vi "EditOptions.vi"(8 "error in":errorcluster, 11 "node in":refnum<class "CustomDevice.lvclass">) -> (0 "error out":errorcluster, 1 "edit options":T1, 2 "subnodes class":T2, 3 "node out":refnum<class "CustomDevice.lvclass">)   [LabVIEW 2019, in "CustomDevice.lvclass"]
doc: "Contains the options for the Menu that will be displayed when doing right click on an item.\nThe sub nodes class configures which nodes can be added to this nodes\nAnd the edit options determine which options are available for the node.\nThis configuration is stored in this VI in case some dynamic configuration is required for the menu options or sub nodes."
uses:
  CustomDevice.lvclass
  C:/Program Files (x86)/National Instruments/LabVIEW 2019/vi.lib/NI/Configuration Framework/Node/NISE_CEF_Node.lvclass
  <vilib>/NI/Configuration Framework/Node/SubNodeCluster.ctl
  <vilib>/NI/Configuration Framework/Node/NodeMenuOptions.ctl
  <vilib>/NI/Configuration Framework/Node/NISE_CEF_Node.lvclass/NISE_CEF_Node.ctl
  <vilib>/NI/Configuration Framework/Node/ReadChildren.vi
  <vilib>/NI/Configuration Framework/Node/ReadNodeClass.vi
  <vilib>/NI/Configuration Framework/Node/NISE_CEF_Node.lvclass
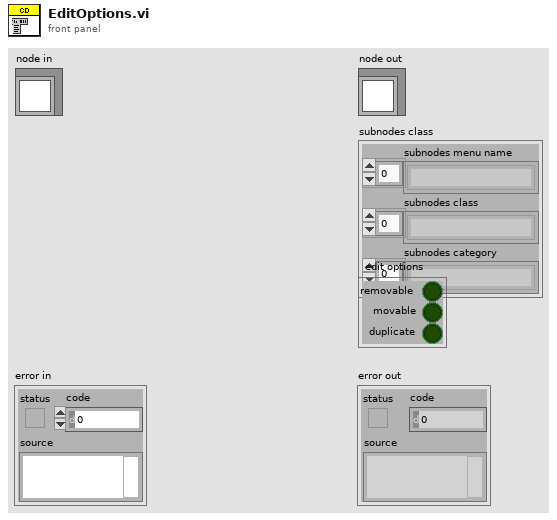
[diagram p1: front panel]
types:
  T1 = typedef "NISE_CEF_Node.lvclass/NodeMenuOptions.ctl" = cluster{"removable":bool, "movable":bool, "duplicate":bool}
  T2 = typedef "NISE_CEF_Node.lvclass/SubNodeCluster.ctl" = cluster{"subnodes menu name":string[], "subnodes class":string[], "subnodes category":string[]}
  T3 = typedef "NISE_CEF_Node.lvclass/NodeRef.ctl" = refnum<data-value>
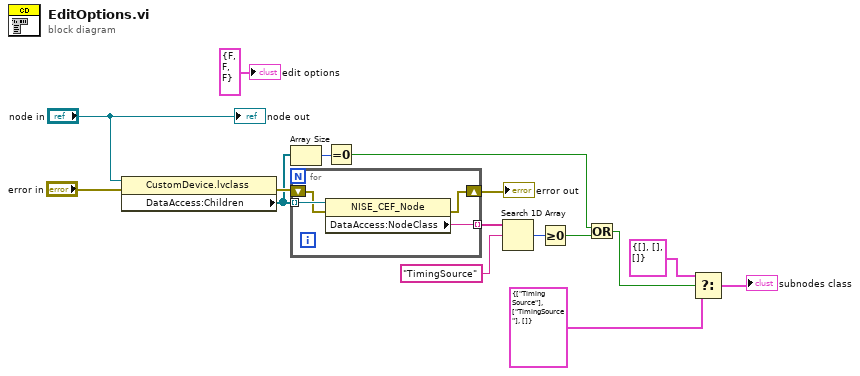
[diagram p0: block diagram]
diagram:
  n1 = property class="CustomDevice.lvclass"(reference="node in", error in="error in") -> (error out=w13:errorcluster, "DataAccess:Children"=w5:T3[])  [unwired: 1 out]
  n2 = Array Size(array=w5) -> (size(s)=w4:i32)
  n3 = for {
    tunnel: w5 -> [w20] mode=indexing
    tunnel: [w19] -> w14 mode=indexing
    shift-right: [w17] -> w12
    shift-left: w13 -> [w18]
    n4 = property class="NISE_CEF_Node"(reference=w20, error in=w18) -> (error out=w17:errorcluster, "DataAccess:NodeClass"=w19:string)  [unwired: 1 out]
  }
  "error out" <- w12
  n5 = Equal To 0?(x=w4) -> (x = 0?=w2:bool)
  n6 = Search 1D Array(1D array=w14, element="TimingSource") -> (index of element=w9:i32)  [unwired: 1 in]
  n7 = Greater Or Equal To 0?(x=w9) -> (x >= 0?=w3:bool)
  n8 = Or(x=w2, y=w3) -> (x .or. y?=w1:bool)
  n9 = Select(t=T2 {"subnodes menu name"=[], "subnodes class"=[], "subnodes category"=[]} ("subnodes class"), s=w1, f=T2 {"subnodes menu name"=["Timing Source"], "subnodes class"=["TimingSource"], "subnodes category"=[]}) -> (s? t:f=→"subnodes class":T2)
  "node out" <- "node in"
  "edit options" <- T1 {"removable"=FALSE, "movable"=FALSE, "duplicate"=FALSE} ("edit options")
